vi "PH_DIM.get Boolean.vi"(1 "no link":bool, 2 "typeDescriptor":string, 3 "data":i8[](array[numeric]), 4 "quality":i32) -> (0 "Value":i32)   [LabVIEW 2014, in "PH_Common.lvlib"]
doc: "This VI calculates the status of Boolean tags. It gives out:\n\n0: no link or wrong data type or tag status bad\n1: link and data type and tag status ok, value = false\n2: link and data type and tag status ok, value = true"
uses:
  PH_Common.lvlib
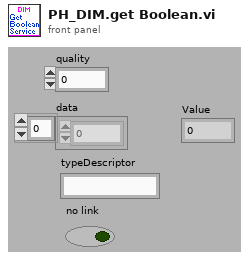
[diagram p1: front panel]
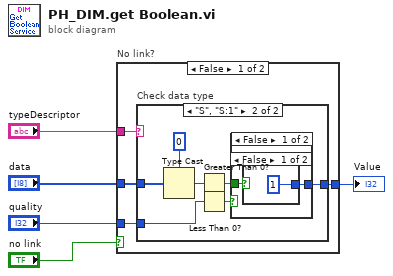
[diagram p0: block diagram]
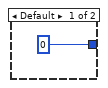
[diagram p2: hidden frame]
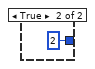
[diagram p3: hidden frame]
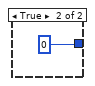
[diagram p4: hidden frame]
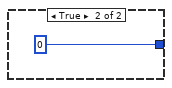
[diagram p5: hidden frame]
diagram:
  n1 = case "No link?" shown="False" "no link" {
    tunnel: [w9 0] -> w5
    tunnel: "quality" -> [w8 _]
    tunnel: "data" -> [w7 _]
    tunnel: "typeDescriptor" -> [w6 _]
    frame False {
      n2 = case "Check data type" shown="\"S\", \"S:1\"" w6 {
        tunnel: [0 w17] -> w9
        tunnel: w8 -> [_ w14]
        tunnel: w7 -> [_ w12]
        frame Default {
        }
        frame "S", "S:1" {
          n3 = Type Cast(type=i16 0, x=w12) -> (*(type *) &x=w11:i16)
          n4 = Greater Than 0?(x=w11) -> (x > 0?=w16:bool)
          n5 = Less Than 0?(x=w14) -> (x < 0?=w15:bool)
          n6 = case shown="False" w15 {
            tunnel: w16 -> [w19 _]
            tunnel: [w18 0] -> w17
            frame False {
              n7 = case shown="False" w19 {
                tunnel: [1 2] -> w18
                frame False {
                }
                frame True {
                }
              }
            }
            frame True {
            }
          }
        }
      }
    }
    frame True {
    }
  }
  "Value" <- w5
